vi "FTW-STR-Repeat.vi"(0 "Times to Repeat":i32=4, 1 "String to Repeat":string=" ") -> (2 "Indented String":string)   [LabVIEW 2012]
panel:
  # "Inputs"
  # "Outputs"
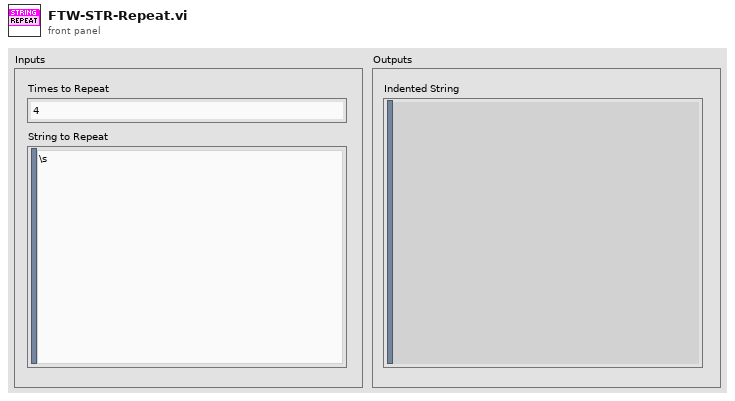
[diagram p1: front panel]
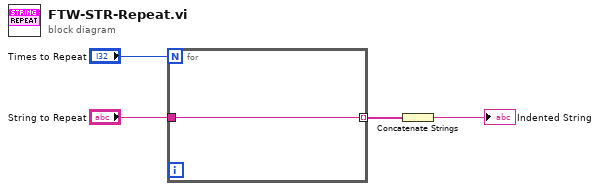
[diagram p0: block diagram]
diagram:
  n1 = for {
    N: "Times to Repeat" -> [_]
    tunnel: "String to Repeat" -> [w5]
    tunnel: [w5] -> w2 mode=indexing
  }
  n2 = Concatenate Strings(w2) -> (→"Indented String":string)
